vi "RPC_DAQV3_mini.vi"(7 "address":string[](array[string])=["192.168.10.20", "192.168.10.35"], 8 "error in (no error)":errorcluster, 9 "stop":bool=TRUE, 11 "SMA mode":bool) -> (0 "error out 3":errorcluster, 2 "csv path":path=path "G:/tdc/2017/data/test_20250827_105458.csv")   [LabVIEW 2017]
uses:
  gloabal.vi
  <vilib>/Utility/file.llb/Write Delimited Spreadsheet (DBL).vi
panel:
  in  "SaveData":bool=TRUE
  out "数组":errorcluster[](array[cluster])
  out "大小 5":i32=2
  out "大小 4":i32=2
  in  "cpu":i32=7
  out "大小 3":i32=2
  out "大小 2":i32=2
  out "大小":i32=2
  out "Array":string[](array[string])
  in  "calib_file":path=path "G:/tdc/2017/data/112_20250410_codeDensity.csv" caption="文件路径 （空时为对话框）"
  in  "use_calib_file":bool
  in  "coarse counter width":u16(ring) items=["29", "48"]
  out "error out 5":errorcluster
  in  "timeout":dbl=30000.0
  out "Out":u8=3 format="%.0x"
  in  "factor":i32=128
  in  "displayCR":bool=TRUE
  in  "Counter Setting":dbl=100000.0 format="%#_13g"
  out "element":string
  in  "UDP Config":bool
  in  "data  path":path=path "G:/tdc/2017/data"
  in  "Thresholds (mV)":dbl[](array[numeric])=[580.0, 580.0, 580.0, 580.0, 600.0, 600.0, 600.0, 600.0, 580.0, 580.0, 600.0, 600.0, 600.0, 600.0, 600.0, 600.0, 580.0, 580.0, 600.0, 600.0, 600.0, 600.0, 600.0, 600.0, 580.0, 580.0, 600.0, 600.0, 600.0, 600.0, 600.0, 600.0, 600.0, 600.0, 600.0, 600.0, 600.0, 600.0, 600.0, 600.0, 600.0, 600.0, 600.0, 600.0, 600.0, 600.0, 600.0, 600.0, 600.0, 600.0, 600.0, 600.0, 600.0, 600.0, 600.0, 600.0, 600.0, 600.0, 600.0, 600.0, 600.0, 600.0, 600.0, 600.0]
  out "error out 2":errorcluster
  in  "display":bool=TRUE
  in  "Thresholds":dbl=-0.03
  in  "one key for threshold":bool=TRUE
  in  "通道数量":i32=10
  out "Event index":i32=97959
  out "error out":errorcluster
  out "appended path":path=path "G:/tdc/2017/data/test_20250827_105458.dat"
  in  "filename":string="test"
  in  "Events":i32=110000 min=1
  in  "timeout (ms)":i32=10000
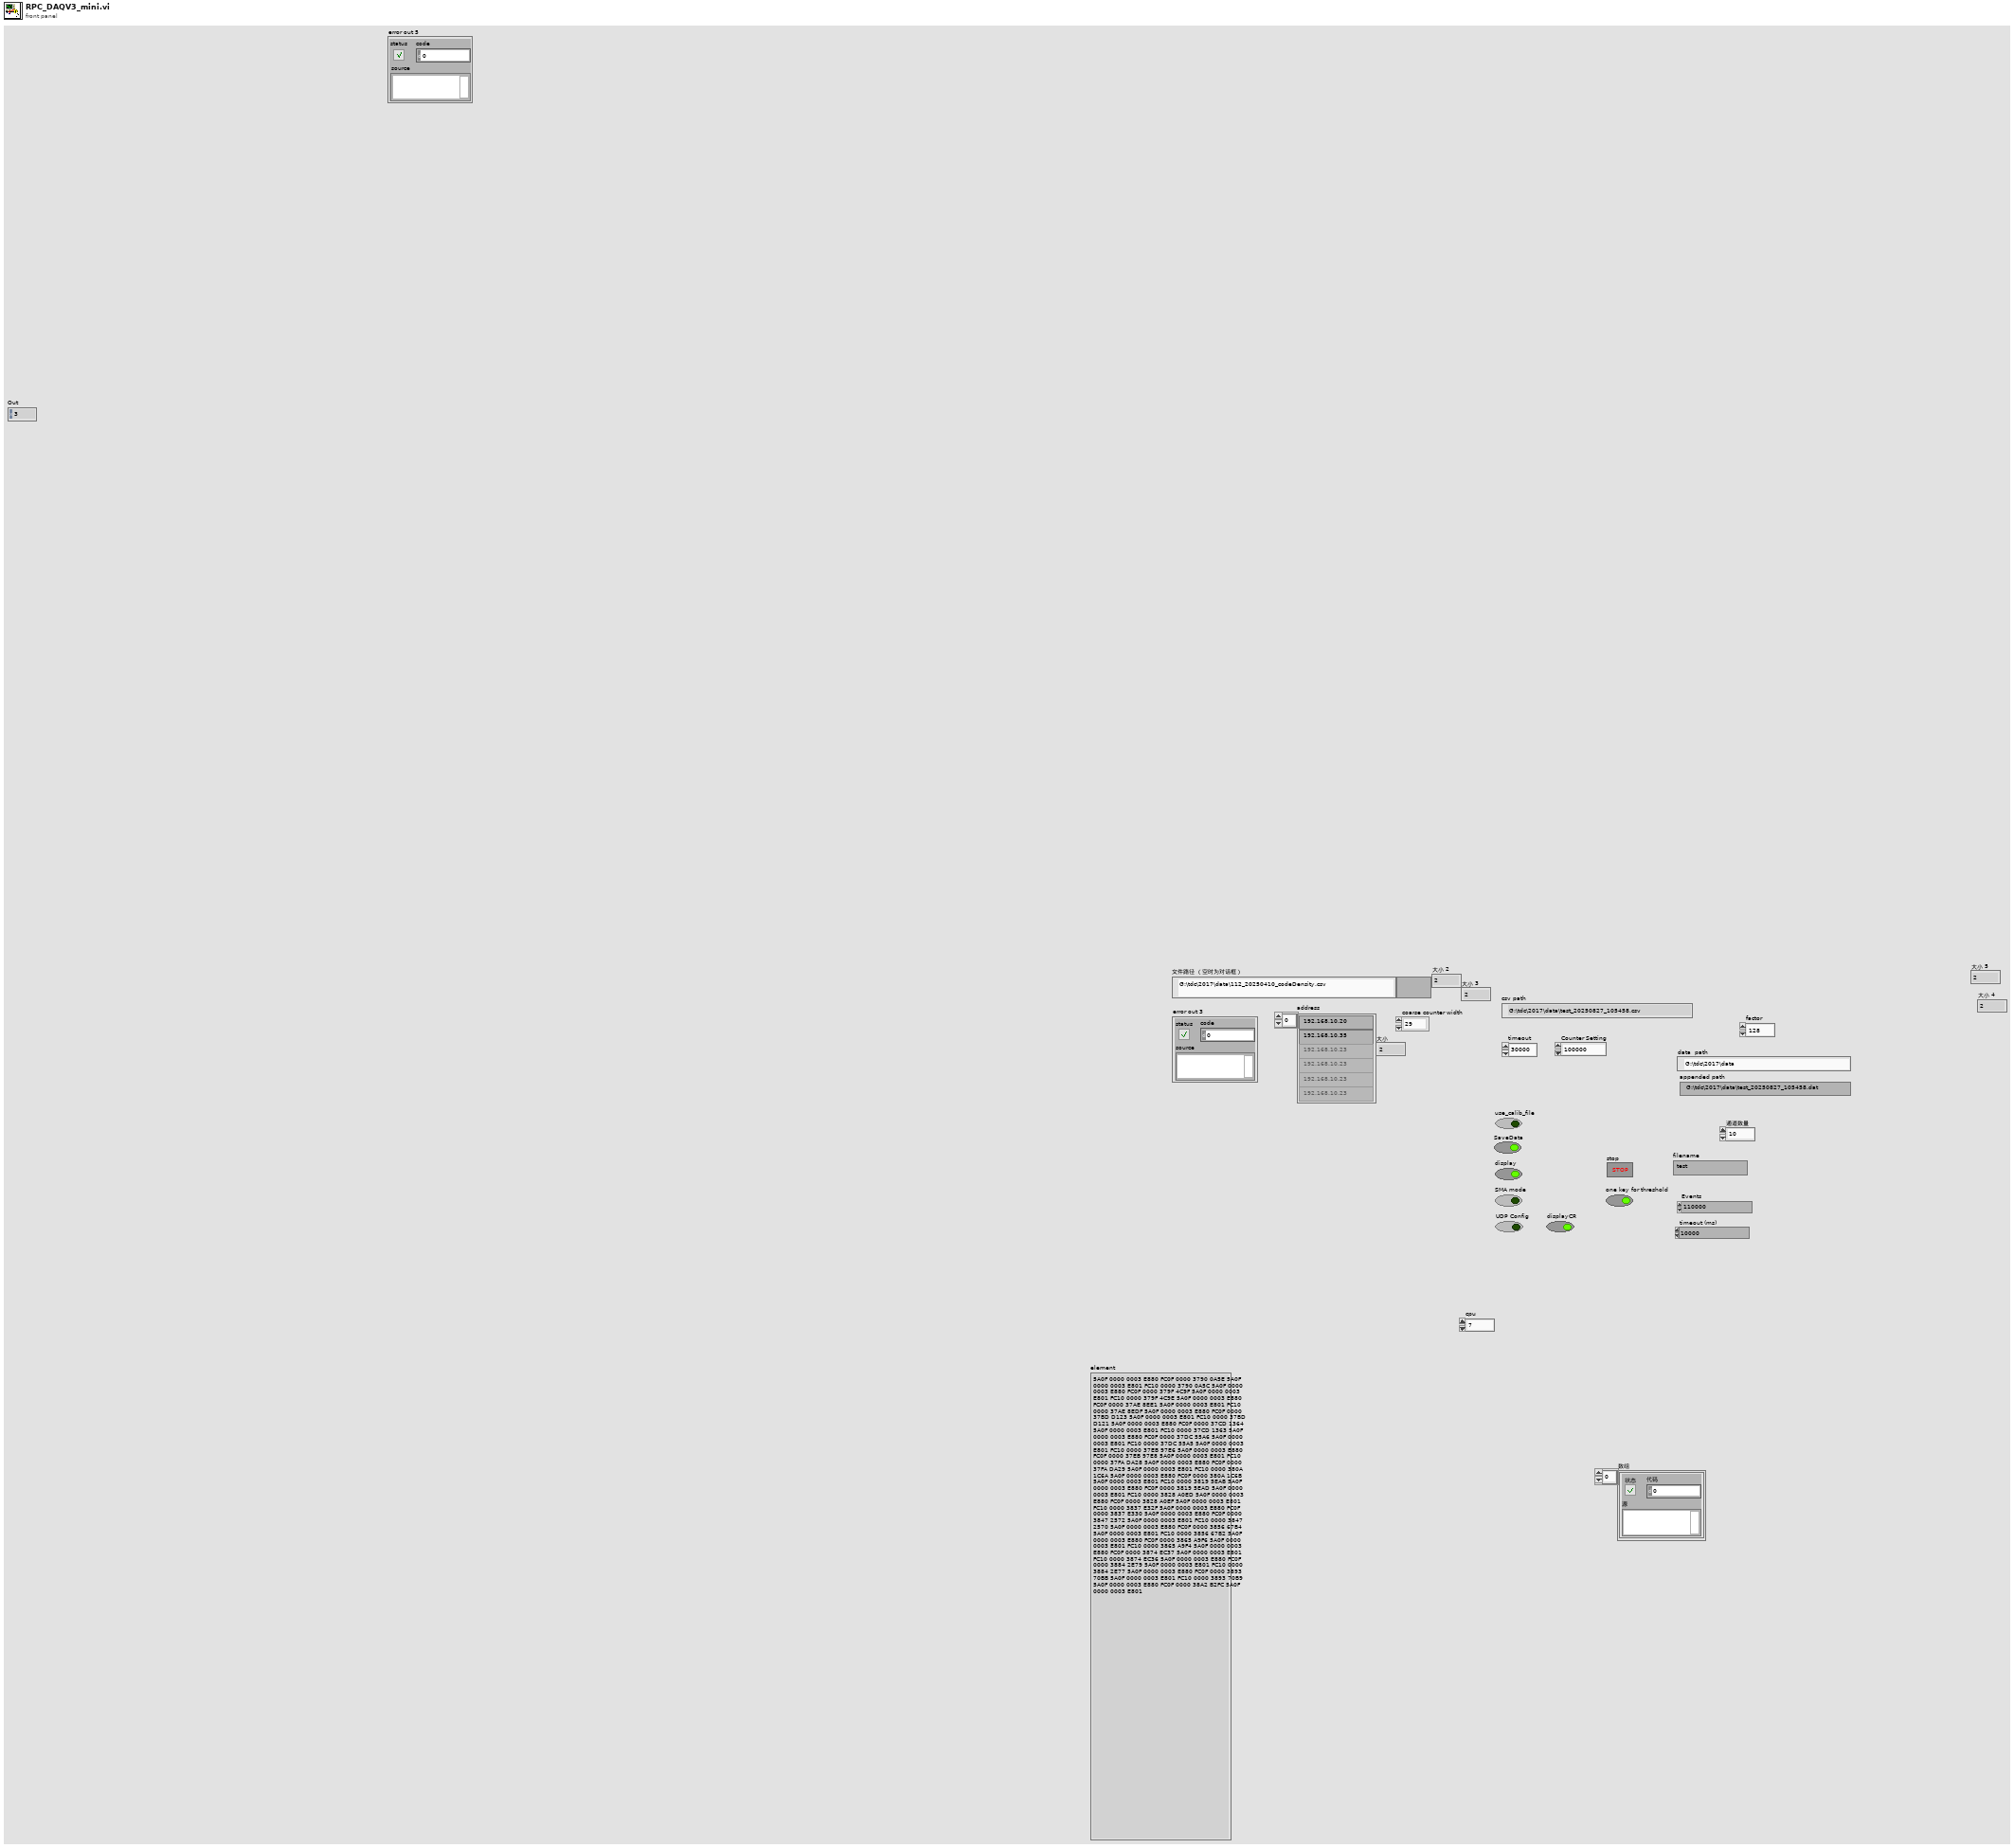
[diagram p1: front panel]
types:
  T1 = enum16{"open", "replace", "create", "open or create", "replace or create", "replace or create with confirmation"}
  T2 = enum16{"big-endian, network order", "native, host order", "little-endian"}
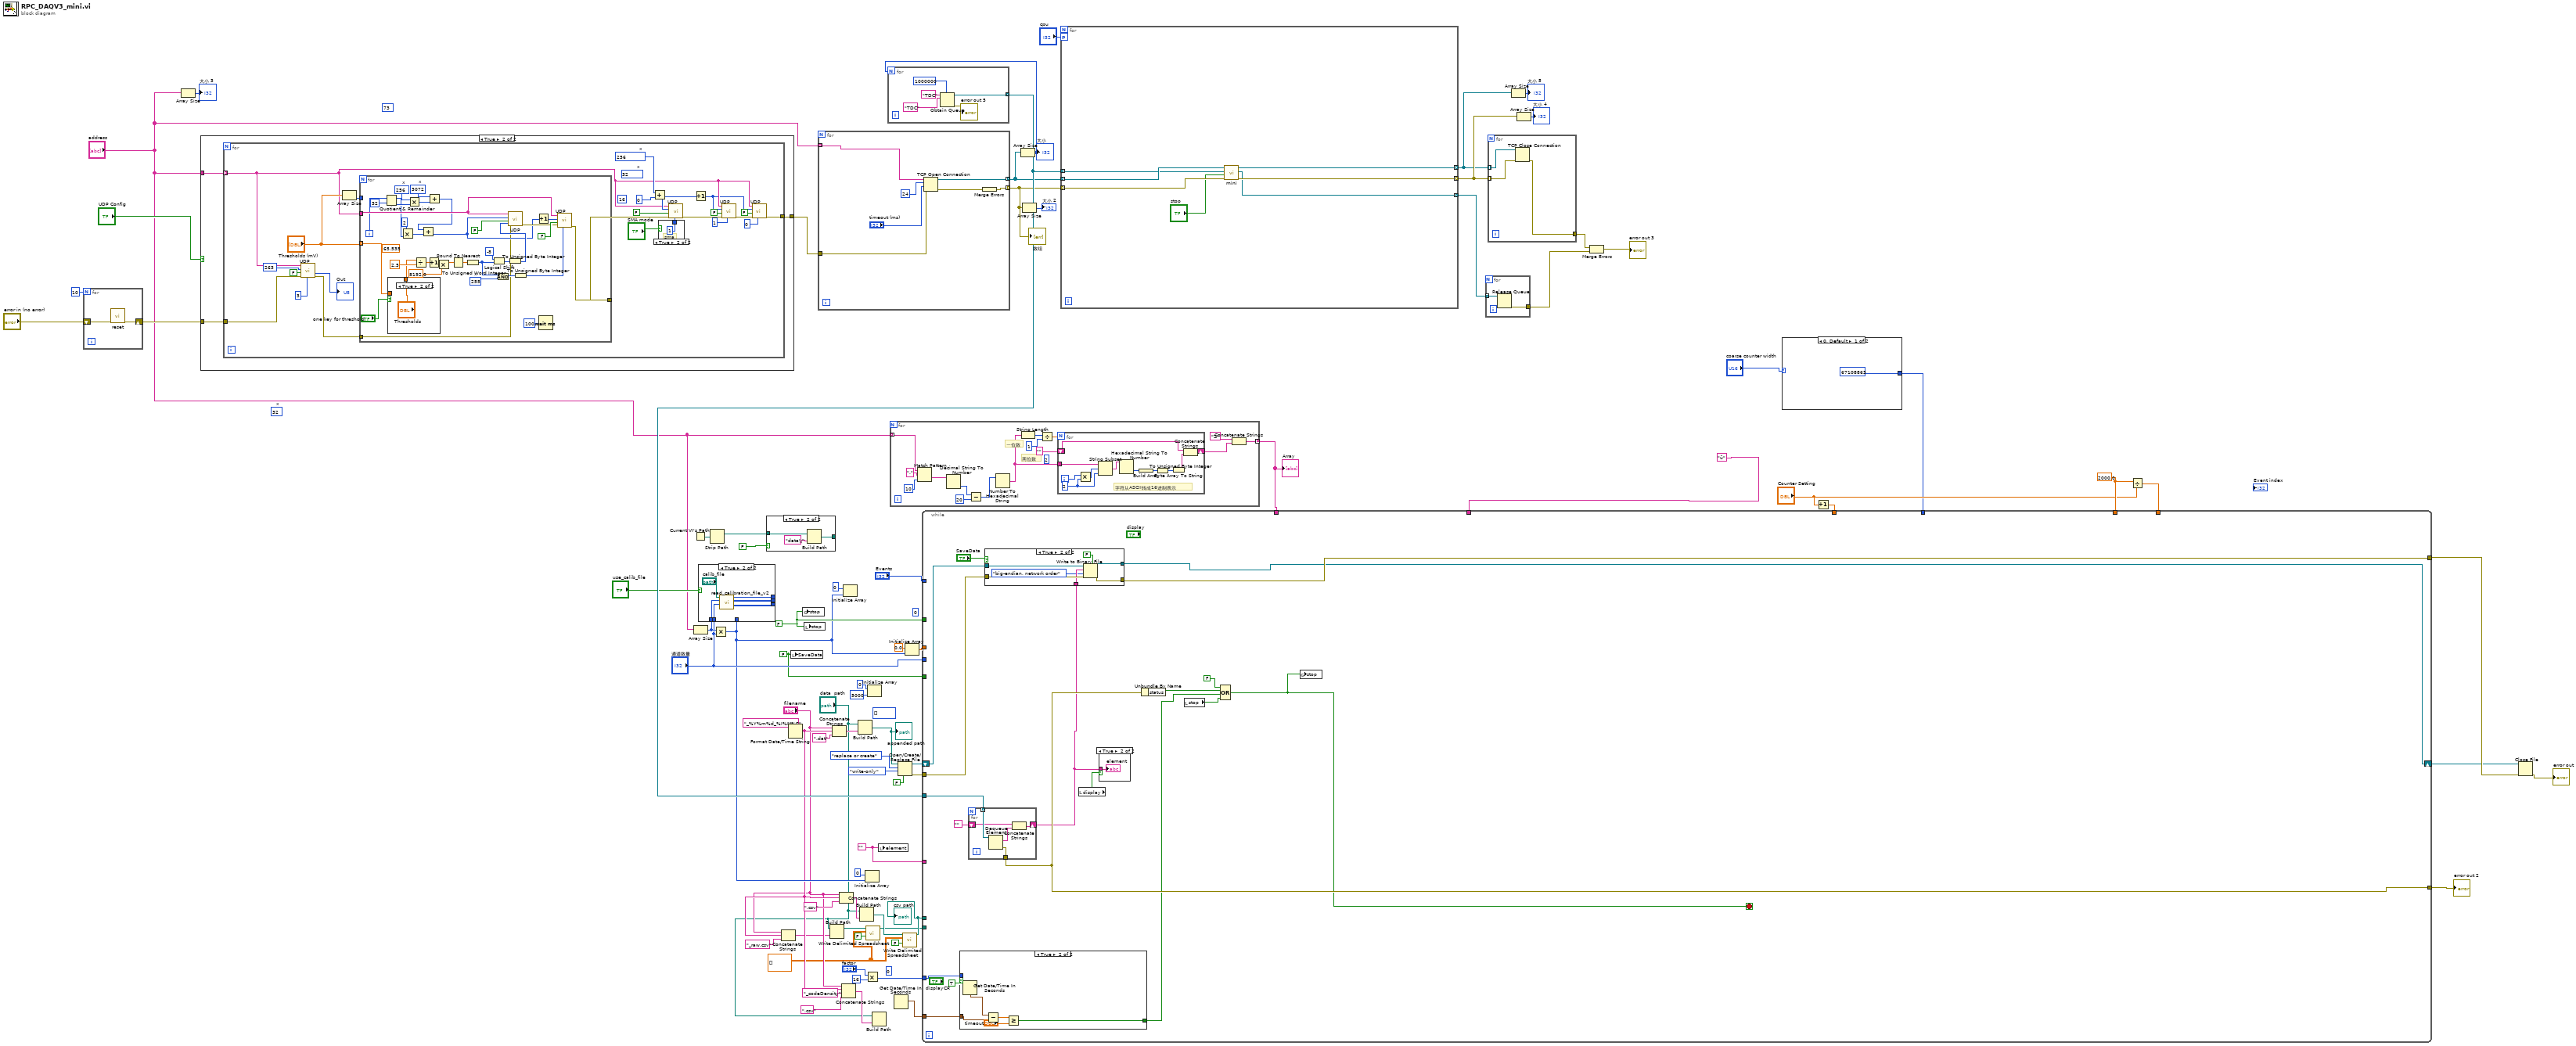
[diagram p0: block diagram]
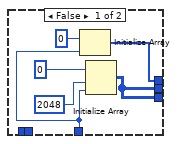
[diagram p2: hidden frame]
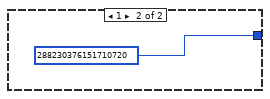
[diagram p3: hidden frame]
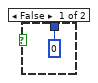
[diagram p5: hidden frame]
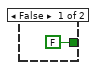
[diagram p10: hidden frame]
diagram:
  w2 = FALSE ("SaveData")
  (unwired) u64[] []
  w25 = ""
  (unwired) u32 73 ("Address")
  w51 = 2000.0 ("x")
  (unwired) u32 0 ("element")
  (unwired) u16 32  # x
  w34 = FALSE ("stop")
  (unwired) 0
  w19 = dbl[][] [] ("2D data")
  n1 = for {
    N: 10 -> [_]
    shift-right: [w81] -> w14
    shift-left: "error in (no error)" -> [w82]
    n2 = call "reset.vi"("error in (no error)"=w82) -> ("error out"=w81:errorcluster)  [unwired: 10 in]
  }
  n3 = Array Size(array="address") -> (size(s)=→"大小 3":i32)
  n4 = case shown="True" "UDP Config" {
    tunnel: "address" -> [_ w84]
    tunnel: [_ w85] -> w38
    tunnel: w14 -> [_ w83]
    frame False {
    }
    frame True {
      n5 = for {
        tunnel: [w91] -> w85
        tunnel: w84 -> [w89] mode=indexing
        tunnel: w83 -> [w86]
        (unwired) u16 32  # x
        (unwired) u32 16 ("Address")
        w102 = u16 256  # x
        n6 = call "UDP.vi"("In"=u8 3, "error in (no error)"=w86, "Read (TRUE)"=FALSE, "Address"=u32 263, "IP address"=w89) -> ("error out"=w97:errorcluster, "Out"=→"Out":u8)  [unwired: 3 in, 1 out]
        n7 = Array Size(array="Thresholds (mV)") -> (size(s)=w105:i32)
        n8 = for {
          tunnel: w89 -> [w141]
          tunnel: "Thresholds (mV)" -> [w128] mode=indexing
          tunnel: [w131] -> w108
          tunnel: w105 -> [_]
          tunnel: w97 -> [w115]
          i -> [w123]
          (unwired) 65.535 ("y")
          w124 = u16 3072  # x
          w125 = u16 256  # x
          w137 = u16 255  # x
          n9 = Quotient & Remainder(x=w123, y=32) -> (x-y*floor(x/y)=w117:i32, floor(x/y)=w126:i32)
          n10 = case shown="True" "one key for threshold" {
            tunnel: [w147 "Thresholds"] -> w129
            tunnel: w128 -> [w147 _]
            frame False {
            }
            frame True {
            }
          }
          n11 = Multiply(x=2, y=w117) -> (x*y=w118:i32)
          n12 = Multiply(x=w125, y=w126) -> (x*y=w120:i32)
          n13 = Divide(x=w129, y=2.5) -> (x/y=w144:dbl)
          n14 = Increment(x=w144) -> (x+1=w114:dbl)
          n15 = Add(x=w124, y=w120) -> (x+y=w119:i32)
          n16 = Add(x=w119, y=w118) -> (x+y=w122:i32)
          n17 = Multiply(x=w114, y=8192.0) -> (x*y=w113:dbl)
          n18 = Round To Nearest(number=w113) -> (nearest integer value=w142:dbl)
          n19 = To Unsigned Word Integer(number=w142) -> (unsigned 16bit integer=w133:u16)
          n20 = Logical Shift(y=i16 -8, x=w133) -> (x << y=w139:u16)
          n21 = And(x=w133, y=w137) -> (x .and. y?=w136:u16)
          n22 = To Unsigned Byte Integer(number=w139) -> (unsigned 8bit integer=w138:u8)
          n23 = call "UDP.vi"("In"=w138, "error in (no error)"=w115, "Read (TRUE)"=FALSE, "Address"=w122, "IP address"=w141) -> ("error out"=w132:errorcluster)  [unwired: 3 in, 2 out]
          n24 = To Unsigned Byte Integer(number=w136) -> (unsigned 8bit integer=w135:u8)
          n25 = Increment(x=w122) -> (x+1=w121:i32)
          n26 = Wait (ms)(milliseconds to wait=u32 100) -> ()  [unwired: 1 out]
          n27 = call "UDP.vi"("In"=w135, "error in (no error)"=w132, "Read (TRUE)"=FALSE, "Address"=w121, "IP address"=w141) -> ("error out"=w131:errorcluster)  [unwired: 3 in, 2 out]
        }
        n28 = Add(x=w102, y=u32 0 ("Address")) -> (x+y=w95:u32)
        n29 = case shown="True" "SMA mode" {
          tunnel: [u8 0 ("In") u8 1 ("In")] -> w107
          frame False {
          }
          frame True {
            # "sma"
          }
        }
        n30 = call "UDP.vi"("In"=w107, "error in (no error)"=w108, "Read (TRUE)"=FALSE, "Address"=w95, "IP address"=w89) -> ("error out"=w96:errorcluster)  [unwired: 3 in, 2 out]
        n31 = Increment(x=w95) -> (x+1=w88:u32)
        n32 = call "UDP.vi"("In"=u8 1, "error in (no error)"=w96, "Read (TRUE)"=FALSE, "Address"=w88, "IP address"=w89) -> ("error out"=w92:errorcluster)  [unwired: 3 in, 2 out]
        n33 = call "UDP.vi"("In"=u8 0, "error in (no error)"=w92, "Read (TRUE)"=FALSE, "Address"=w88, "IP address"=w89) -> ("error out"=w91:errorcluster)  [unwired: 3 in, 2 out]
      }
    }
  }
  n34 = Current VI's Path() -> (path=w75:path)
  n35 = Array Size(array="address") -> (size(s)=w29:i32)
  n36 = Strip Path(path=w75) -> (stripped path=w74:path)  [unwired: 1 out]
  n37 = Multiply(x=w29, y="通道数量") -> (x*y=w26:i32)
  n38 = case shown="True" "use_calib_file" {
    tunnel: w26 -> [w152 _]
    tunnel: [w149 w160] -> _
    tunnel: [w149 w159] -> _
    tunnel: [w150 w158] -> _
    tunnel: w29 -> [_ w157]
    tunnel: "通道数量" -> [_ w156]
    frame False {
      n39 = Initialize Array(u32 0 ("element"), w152) -> (w150:u32[])
      n40 = Initialize Array(u32 0 ("element"), 2048 ("dimension size"), w152) -> (w149:u32[][])
    }
    frame True {
      n41 = call "read_calibration_file_v2.vi"("通道数量"=w156, "板子数量"=w157, "file path (dialog if empty)"="calib_file") -> ("code_density"=w160:i64[][], "accumulation"=w159:u32[][], "Cal Table"=w158:u32[])  [unwired: 5 in, 1 out]
    }
  }
  n42 = case shown="True" FALSE {
    tunnel: w74 -> [w161 w163]
    tunnel: [w161 w162] -> _
    frame False {
    }
    frame True {
      n43 = Build Path(base path=w163, name or relative path="data\\") -> (appended path=w162:path)
    }
  }
  n44 = Format Date/Time String(time format string (%c)="_%Y%m%d_%I%M%S") -> (date/time string=w23:string)  [unwired: 2 in]
  n45 = Concatenate Strings("filename", w23, "_raw.csv") -> (w21:string)
  n46 = local write "SaveData"(w2) -> ()
  n47 = global write "gloabal.vi" "stop"(w34) -> ()
  n48 = local write "stop"(w34) -> ()
  n49 = for {
    tunnel: "address" -> [w170] mode=indexing
    tunnel: [w169] -> w12 mode=indexing
    tunnel: [w167] -> w13 mode=indexing
    tunnel: w38 -> [w166]
    n50 = TCP Open Connection(address=w170, remote port or service name=u16 24 ("port"), timeout ms (60000)="timeout (ms)", error in (no error)=w166) -> (connection ID=w169:refnum<k5>, error out=w168:errorcluster)  [unwired: 1 in]
    n51 = Merge Errors(w168) -> (w167:errorcluster)
  }
  "数组" <- w13
  n52 = Build Path(base path="data  path", name or relative path=w21) -> (appended path=w16:path)
  n53 = Concatenate Strings("filename", w23, ".dat") -> (w73:string)
  n54 = Concatenate Strings("filename", w23, ".csv") -> (w63:string)
  n55 = Concatenate Strings("filename", w23, "_codeDensity" ("string"), ".csv") -> (w57:string)
  n56 = Initialize Array(u32 0 ("element"), w26) -> ()  [unwired: 1 out]
  n57 = Build Path(base path="data  path", name or relative path=w73) -> (appended path=w72:path)
  "appended path" <- w72
  n58 = Build Path(base path="data  path", name or relative path=w63) -> (appended path=w62:path)
  n59 = Initialize Array(u32 0 ("element"), w26) -> ()  [unwired: 1 out]
  n60 = call-poly <vilib>:"Write Delimited Spreadsheet.vi"("file path (dialog if empty)"=w16, "2D data"=w19, "append to file? (new file:F)"=FALSE) -> ("new file path (Not A Path if cancelled)"=w17:path)  [unwired: 11 in, 1 out]
  n61 = Multiply(x="factor", y=16) -> (x*y=w45:i32)
  n62 = Initialize Array(u32 0 ("element"), 5000 ("dimension size")) -> ()  [unwired: 1 out]
  n63 = Build Path(base path="data  path", name or relative path=w57) -> ()  [unwired: 1 out]
  n64 = local write "element"(w25) -> ()
  n65 = for {
    tunnel: [w173] -> w42 mode=indexing
    tunnel: "address" -> [w172] mode=indexing
    (unwired) 2 ("y")
    # "一位数"
    # "两位数"
    n66 = Match Pattern(string=w172, regular expression="." ("search string"), offset (0)=10) -> (after substring=w179:string)  [unwired: 3 out]
    n67 = Decimal String To Number(string=w179) -> (number=w176:i32)  [unwired: 2 in, 1 out]
    n68 = Subtract(x=w176, y=20) -> (x-y=w175:i32)
    n69 = Number To Hexadecimal String(2:w175) -> (0:w178:string)  [unwired: 1 in]
    n70 = String Length(string=w178) -> (length=w184:i32)
    n71 = Divide(x=w184, y=1) -> (x/y=w185:dbl)
    n72 = for {
      N: w185 -> [_]
      shift-right: [w197] -> w174
      shift-left: "" ("format string") -> [w196]
      tunnel: w178 -> [w187]
      i -> [w195]
      w189 = 2 ("y")
      # "字符从ASCII转成16进制表示"
      n73 = Multiply(x=w195, y=w189) -> (x*y=w188:i32)
      n74 = String Subset(string=w187, offset (0)=w188, length (rest)=w189) -> (substring=w190:string)
      n75 = Hexadecimal String To Number(string=w190) -> (number=w194:u32)  [unwired: 2 in, 1 out]
      n76 = Build Array(w194) -> (w193:u32[])
      n77 = To Unsigned Byte Integer(number=w193) -> (unsigned 8bit integer=w192:u8[])
      n78 = Byte Array To String(unsigned byte array=w192) -> (string=w191:string)
      n79 = Concatenate Strings(w196, w191) -> (w197:string)
    }
    n80 = Concatenate Strings("Z", w174) -> (w173:string)
  }
  "Array" <- w42
  n81 = Get Date/Time In Seconds() -> (seconds since 1Jan1904=w41:timestamp)
  n82 = Open/Create/Replace File(file path (use dialog)=w72, operation (0:open)=T1."replace or create", access (0:read/write)=enum16{"read/write", "read-only", "write-only"}."write-only", disable buffering (F)=FALSE) -> (refnum out=w77:refnum<file>, error out=w76:errorcluster)  [unwired: 2 in, 1 out]
  n83 = call-poly <vilib>:"Write Delimited Spreadsheet.vi"("file path (dialog if empty)"=w62, "2D data"=w19, "append to file? (new file:F)"=FALSE) -> ("new file path (Not A Path if cancelled)"=w33:path)  [unwired: 11 in, 1 out]
  "csv path" <- w33
  n84 = Initialize Array(0.0, w26) -> (w55:dbl[])
  n85 = Array Size(array=w12) -> (size(s)=w4:i32)
  "大小" <- w4
  n86 = for {
    N: w4 -> [_]
    tunnel: [w198] -> w39 mode=indexing
    n87 = Obtain Queue(max queue size (-1, unlimited)=1000000, name (unnamed)="TDC", element data type="TDC" ("name (unnamed)")) -> (queue out=w198:refnum<queue>, error out=→"error out 5":errorcluster)  [unwired: 2 in, 1 out]
  }
  n88 = Array Size(array=w13) -> (size(s)=→"大小 2":i32)
  n89 = for {
    tunnel: w12 -> [w209] mode=indexing
    tunnel: w13 -> [w208] mode=indexing
    tunnel: [w207] -> w5 mode=indexing
    tunnel: [w206] -> w7 mode=indexing
    tunnel: w39 -> [w205] mode=indexing
    tunnel: [w204] -> w40 mode=indexing
    workers-P: "cpu" -> [_]
    n90 = call "mini.vi"("error in (no error)"=w208, "stop"="stop", "queue out 2"=w205, "connection ID 2"=w209) -> ("error out 3"=w206:errorcluster, "queue out"=w204:refnum<queue>, "connection ID"=w207:refnum<k5>)  [unwired: 5 in]
  }
  n91 = for {
    tunnel: w40 -> [w211] mode=indexing
    tunnel: [w210] -> w36
    n92 = Release Queue(queue=w211) -> (error out=w210:errorcluster)  [unwired: 2 in, 2 out]
  }
  n93 = for {
    tunnel: w5 -> [w214] mode=indexing
    tunnel: w7 -> [w213] mode=indexing
    tunnel: [w212] -> w37
    n94 = TCP Close Connection(connection ID=w214, error in (no error)=w213) -> (error out=w212:errorcluster)  [unwired: 1 in, 1 out]
  }
  n95 = Array Size(array=w5) -> (size(s)=→"大小 5":i32)
  n96 = Array Size(array=w7) -> (size(s)=→"大小 4":i32)
  n97 = Merge Errors(w37, w36) -> (→"error out 3":errorcluster)
  n98 = case shown="0, Default" "coarse counter width" {
    tunnel: [u64 67108863 ("port") u64 288230376151710720 ("port")] -> w31
    frame 0, Default {
    }
    frame 1 {
    }
  }
  n99 = Increment(x="Counter Setting") -> (x+1=w47:dbl)
  n100 = Divide(x=w51, y="Counter Setting") -> (x/y=w50:dbl)
  n101 = while {
    tunnel: w76 -> [w234]
    tunnel: [w231] -> w56
    tunnel: [w228] -> w69
    tunnel: "Events" -> [_]
    tunnel: w33 -> [_]
    tunnel: w34 -> [_]
    tunnel: w39 -> [w232]
    tunnel: w42 -> [_]
    tunnel: w51 -> [_]
    tunnel: w50 -> [_]
    shift-right: [w227] -> w49
    shift-left: w77 -> [w233]
    tunnel: w47 -> [_]
    tunnel: w45 -> [w225]
    tunnel: "ü" ("format string") -> [_]
    tunnel: w41 -> [w223]
    tunnel: "通道数量" -> [_]
    tunnel: w31 -> [_]
    tunnel: w25 -> [_]
    tunnel: w17 -> [_]
    tunnel: w55 -> [_]
    tunnel: w2 -> [_]
    stop <- w221 stop-if-true
    n102 = case shown="True" TRUE {
      tunnel: w225 -> [_ _]
      tunnel: w223 -> [_ w254]
      tunnel: [FALSE w251] -> w222
      frame False {
      }
      frame True {
        n103 = Get Date/Time In Seconds() -> (seconds since 1Jan1904=w255:timestamp)
        n104 = Subtract(x=w255, y=w254) -> (x-y=w253:dbl)
        n105 = Greater Or Equal?(x=w253, y="timeout") -> (x >= y?=w251:bool)
      }
    }
    n106 = for {
      tunnel: w232 -> [w239] mode=indexing
      tunnel: [w238] -> w231
      shift-right: [w237] -> w218
      shift-left: "" -> [w235]
      n107 = Dequeue Element(queue=w239) -> (element=w236:string, error out=w238:errorcluster)  [unwired: 2 in, 2 out]
      n108 = Concatenate Strings(w235, w236) -> (w237:string)
    }
    n109 = case shown="True" "SaveData" {
      tunnel: w234 -> [w241 w249]
      tunnel: w233 -> [w242 w248]
      tunnel: w218 -> [_ w246]
      tunnel: [w242 w245] -> w227
      tunnel: [w241 w244] -> w228
      frame False {
      }
      frame True {
        n110 = Write to Binary File(file (use dialog)=w248, data=w246, error in=w249, 5:FALSE ("prepend array or string size? (T)"), 9:T2."big-endian, network order" ("byte order (0:big-endian, network order)")) -> (refnum out=w245:refnum<file>, error out=w244:errorcluster)  [unwired: 1 in, 1 out]
      }
    }
    n111 = local read "display"() -> (w226:bool)
    n112 = case shown="True" w226 {
      tunnel: w218 -> [_ w240]
      frame False {
      }
      frame True {
        "element" <- w240
      }
    }
    n113 = Unbundle By Name(w231) -> ("status"=w230:bool)
    n114 = local read "stop"() -> (w220:bool)
    n115 = Compound Arithmetic op=OR(FALSE ("x"), w230, w222, w220) -> (w221:bool)
    n116 = global write "gloabal.vi" "stop"(w221) -> ()
  }
  "error out 2" <- w56
  n117 = Close File(refnum=w49, error in=w69) -> (error out=→"error out":errorcluster)  [unwired: 1 out]
